vi "ZDS1104 SingleConfig.vi"(8 "错误输入":errorcluster, 9 "Trigger Level":dbl, 10 "Channel":i32(ring)=1 items=["Channel 1"=1, "Channel 2"=2, "Channel 3"=3, "Channel 4"=4], 11 "MyIndex":u8) -> (0 "error out":errorcluster caption="错误输出", 3 "ok?":bool)   [LabVIEW 2015]
uses:
  ZhiYuan ZDS Series for TCP/Public/Configure/Trigger/Configure Trigger (Edge).vi
  ZhiYuan ZDS Series for TCP/ZhiYuan ZDS Series for TCP.lvlib
panel:
  out "VISA":refnum<visa-resource-name> caption="VISA资源名称输出"
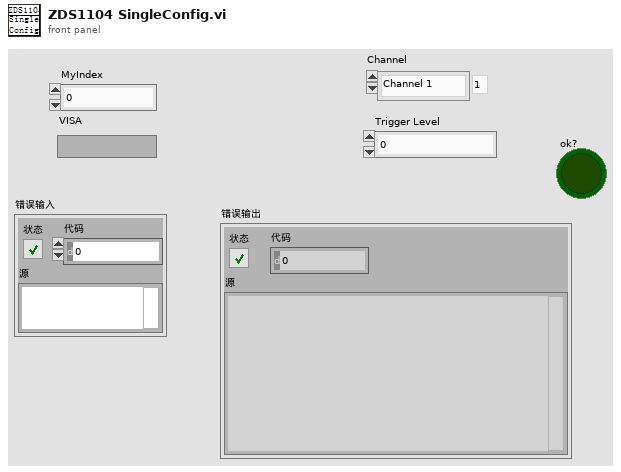
[diagram p1: front panel]
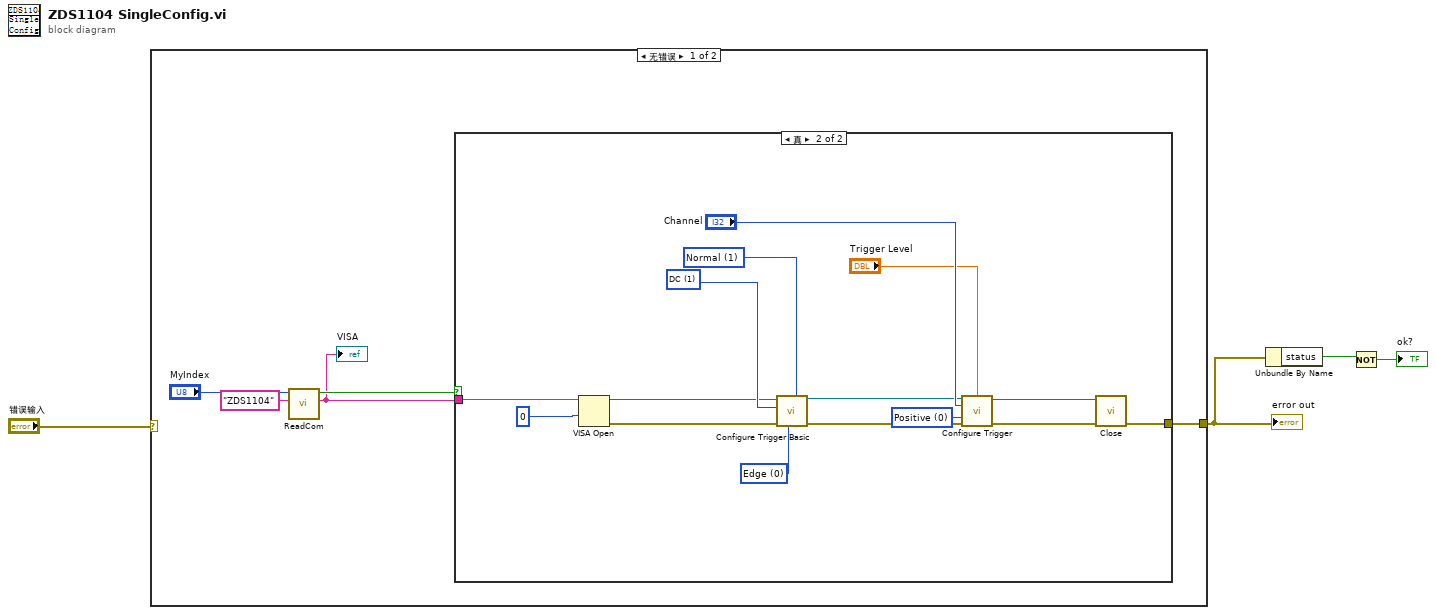
[diagram p0: block diagram]
diagram:
  n1 = case shown="无错误" "错误输入" {
    selector: "错误输入" -> [_ w25]
    tunnel: [w9 w25] -> w2
    frame No Error {
      n2 = call "ReadCom.vi"("仪器名称"="ZDS1104", "MyIndex"="MyIndex") -> ("COM"=w5:string, "OK?"=w6:bool)  [unwired: 7 in, 1 out]
      "VISA" <- w5
      n3 = case shown="真" w6 {
        tunnel: [_ w22] -> w9
        tunnel: w5 -> [_ w23]
        frame False {
        }
        frame True {
          w21 = 0 items=["Edge", "Pulse", "Slope", "Video", "Runt", "Prunt", "Pattern", "Nth Edge", "Delay", "Timeout", "Setup/Hold"] ("Trigger Type (0: Edge)")
          w20 = 1 items=["AC", "DC", "LF Reject", "HF Reject"] ("Coupling Mode (0: AC)")
          w19 = 1 items=["Auto", "Normal"] ("Trigger Mode (0: Auto)")
          w18 = 0 items=["Positive", "Negative", "Either"] ("Edge Type (0: Positive)")
          n4 = VISA Open(access mode=u32 0, VISA resource name=w23) -> (VISA resource name=w10:refnum<visa-resource-name>, error out=w13:errorcluster)  [unwired: 3 in]
          n5 = call "Configure Trigger Basic.vi"("Trigger Mode (0: Auto)"=w19, "Trigger Type (0: Edge)"=w21, "error in (no error)"=w13, "Coupling Mode (0: AC)"=w20, "VISA resource name"=w10) -> ("error out"=w14:errorcluster, "VISA resource name out"=w15:refnum<visa-resource-name>)  [unwired: 5 in]
          n6 = call-poly "Configure Trigger.vi"("VISA resource name"=w15, "Trigger Level (0)"="Trigger Level", "Source (1: Channel 1)"="Channel", "Edge Type (0: Positive)"=w18, "error in (no error)"=w14) -> ("VISA resource name out"=w11:refnum<visa-resource-name>, "error out"=w12:errorcluster)  [unwired: 9 in]
          n7 = call "Close.vi"("error in (no error)"=w12, "VISA resource name"=w11) -> ("error out"=w22:errorcluster)  [unwired: 9 in]
        }
      }
    }
    frame Error {
    }
  }
  "error out" <- w2
  n8 = Unbundle By Name(w2) -> ("status"=w4:bool)
  n9 = Not(x=w4) -> (.not. x?=→"ok?":bool)
